vi "EXCOM-TCP-25.vi"(0 "connection ID":refnum<k5>, 5 "Error IN":errorcluster) -> (6 "HA":dbl format="%<%H:%M:%S%0u>t", 7 "Q String":string, 8 "RA":dbl format="%<%H:%M:%S%0u>t", 9 "Rotateur":dbl format="%.2f", 10 "DEC":dbl format="%<%H:%M:%S%0u>t", 11 "Dome":dbl format="%.2f", 12 "Epoque":dbl format="%.2f", 13 "Focus":dbl format="%.2f", 14 "CID Out":refnum<k5>, 15 "Masse d'air":dbl format="%.2f", 16 "Temps Sidéral":dbl format="%<%H:%M:%S%0u>t", 17 "Temps Universel":dbl format="%<%H:%M:%S%0u>t", 18 "Année":dbl format="%.2f", 19 "Error Out":errorcluster)   [LabVIEW 2011]
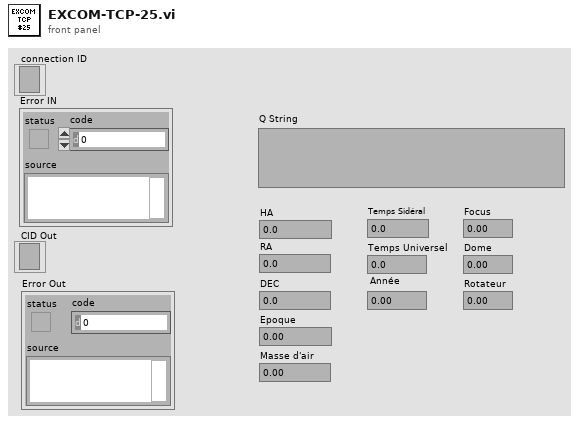
[diagram p1: front panel]
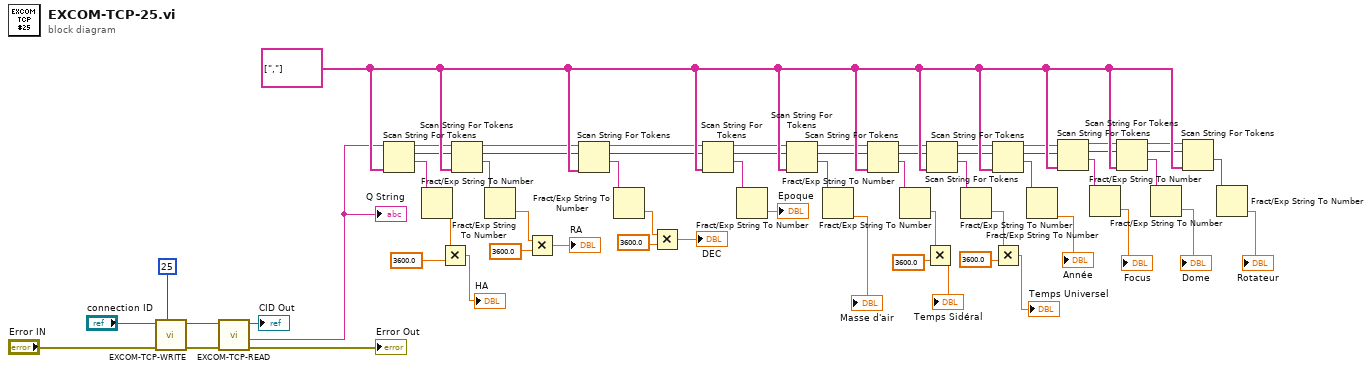
[diagram p0: block diagram]
diagram:
  w55 = string[] [","] ("delimiters (\\s,\\t,\\r,\\n)")
  n1 = call "EXCOM-TCP-WRITE.vi"("Commande #"=25, "Error IN"="Error IN", "connection ID"="connection ID") -> ("Error OUT"=w57:errorcluster, "connection ID out"=w58:refnum<k5>)  [unwired: 4 in, 2 out]
  n2 = call "EXCOM-TCP-READ.vi"("Error In"=w57, "connection ID"=w58) -> ("Error Out"=→"Error Out":errorcluster, "Response"=w3:string, "CID Out"=→"CID Out":refnum<k5>)  [unwired: 5 in]
  "Q String" <- w3
  n3 = Scan String For Tokens(6:w55, 9:w3) -> (1:w12:string, 2:w11:i32, 3:w10:string)  [unwired: 4 in, 1 out]
  n4 = Fract/Exp String To Number(string=w12) -> (number=w13:dbl)  [unwired: 3 in, 1 out]
  n5 = Multiply(x=w13, y=3600.0) -> (x*y=→"HA":dbl)
  n6 = Scan String For Tokens(6:w55, 8:w11, 9:w10) -> (1:w54:string, 2:w8:i32, 3:w9:string)  [unwired: 3 in, 1 out]
  n7 = Fract/Exp String To Number(string=w54) -> (number=w21:dbl)  [unwired: 3 in, 1 out]
  n8 = Multiply(x=w21, y=3600.0) -> (x*y=→"RA":dbl)
  n9 = Scan String For Tokens(6:w55, 8:w8, 9:w9) -> (1:w18:string, 2:w6:i32, 3:w7:string)  [unwired: 3 in, 1 out]
  n10 = Fract/Exp String To Number(string=w18) -> (number=w23:dbl)  [unwired: 3 in, 1 out]
  n11 = Multiply(x=w23, y=3600.0) -> (x*y=→"DEC":dbl)
  n12 = Scan String For Tokens(6:w55, 8:w6, 9:w7) -> (1:w19:string, 2:w4:i32, 3:w5:string)  [unwired: 3 in, 1 out]
  n13 = Fract/Exp String To Number(string=w19) -> (number=→"Epoque":dbl)  [unwired: 3 in, 1 out]
  n14 = Scan String For Tokens(6:w55, 8:w4, 9:w5) -> (1:w20:string, 2:w52:i32, 3:w33:string)  [unwired: 3 in, 1 out]
  n15 = Fract/Exp String To Number(string=w20) -> (number=→"Masse d'air":dbl)  [unwired: 3 in, 1 out]
  n16 = Scan String For Tokens(6:w55, 8:w52, 9:w33) -> (1:w28:string, 2:w30:i32, 3:w29:string)  [unwired: 3 in, 1 out]
  n17 = Fract/Exp String To Number(string=w28) -> (number=w25:dbl)  [unwired: 3 in, 1 out]
  n18 = Multiply(x=w25, y=3600.0) -> (x*y=→"Temps Sidéral":dbl)
  n19 = Scan String For Tokens(6:w55, 8:w30, 9:w29) -> (1:w27:string, 2:w32:i32, 3:w31:string)  [unwired: 3 in, 1 out]
  n20 = Fract/Exp String To Number(string=w27) -> (number=w24:dbl)  [unwired: 3 in, 1 out]
  n21 = Scan String For Tokens(6:w55, 8:w32, 9:w31) -> (1:w26:string, 2:w53:i32, 3:w43:string)  [unwired: 3 in, 1 out]
  n22 = Multiply(x=w24, y=3600.0) -> (x*y=→"Temps Universel":dbl)
  n23 = Fract/Exp String To Number(string=w26) -> (number=→"Année":dbl)  [unwired: 3 in, 1 out]
  n24 = Scan String For Tokens(6:w55, 8:w53, 9:w43) -> (1:w40:string, 2:w38:i32, 3:w39:string)  [unwired: 3 in, 1 out]
  n25 = Fract/Exp String To Number(string=w40) -> (number=→"Focus":dbl)  [unwired: 3 in, 1 out]
  n26 = Scan String For Tokens(6:w55, 8:w38, 9:w39) -> (1:w41:string, 2:w36:i32, 3:w37:string)  [unwired: 3 in, 1 out]
  n27 = Fract/Exp String To Number(string=w41) -> (number=→"Dome":dbl)  [unwired: 3 in, 1 out]
  n28 = Scan String For Tokens(6:w55, 8:w36, 9:w37) -> (1:w42:string)  [unwired: 3 in, 3 out]
  n29 = Fract/Exp String To Number(string=w42) -> (number=→"Rotateur":dbl)  [unwired: 3 in, 1 out]
